vi "temperature_checksum.vi"(1 "Input string":string) -> (0 "Checksum":string)   [LabVIEW 2011]
doc: "moreChemistry's general purpose CRC vi\ncopyright 2004 moreChemistry BART BOSHUIZEN"
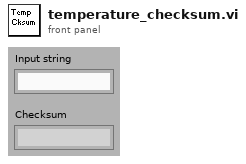
[diagram p1: front panel]
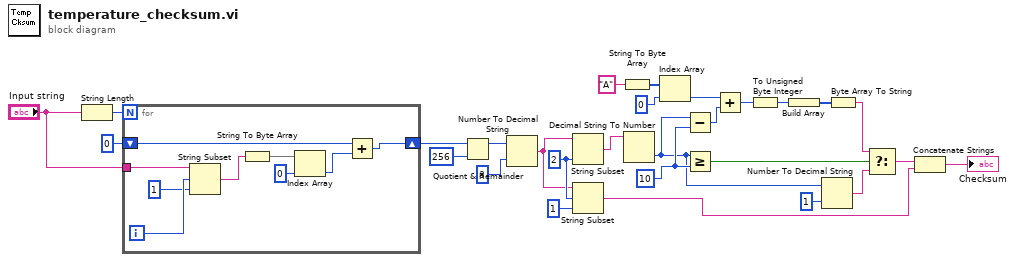
[diagram p0: block diagram]
diagram:
  w16 = 10 ("y")
  w8 = 2 ("length (rest)")
  n1 = String Length(string="Input string") -> (length=w25:i32)
  n2 = for {
    N: w25 -> [_]
    tunnel: "Input string" -> [w37]
    shift-right: [w32] -> w2
    shift-left: i16 0 -> [w30]
    i -> [w36]
    n3 = String Subset(string=w37, offset (0)=w36, length (rest)=1) -> (substring=w34:string)
    n4 = String To Byte Array(string=w34) -> (unsigned byte array=w31:u8[])
    n5 = Index Array(array=w31, index=0) -> (element=w29:u8)
    n6 = Add(x=w30, y=w29) -> (x+y=w32:i16)
  }
  n7 = Quotient & Remainder(x=w2, y=256) -> (x-y*floor(x/y)=w1:i32)  [unwired: 1 out]
  n8 = Number To Decimal String(number=w1, width (-)=i16 3) -> (decimal integer string=w6:string)
  n9 = String Subset(string=w6, length (rest)=w8) -> (substring=w23:string)  [unwired: 1 out]
  n10 = String Subset(string=w6, offset (0)=w8, length (rest)=1 ("length (rest)")) -> (substring=w4:string)
  n11 = String To Byte Array(string="A") -> (unsigned byte array=w18:u8[])
  n12 = Decimal String To Number(string=w23) -> (number=w12:i32)  [unwired: 3 out]
  n13 = Index Array(array=w18, index=0) -> (element=w14:u8)
  n14 = Subtract(x=w12, y=w16) -> (x-y=w15:i32)
  n15 = Greater Or Equal?(x=w12, y=w16) -> (x >= y?=w22:bool)
  n16 = Add(x=w14, y=w15) -> (x+y=w13:i32)
  n17 = To Unsigned Byte Integer(number=w13) -> (unsigned 8bit integer=w21:u8)
  n18 = Build Array(w21) -> (w20:u8[])
  n19 = Number To Decimal String(number=w12, width (-)=i16 1) -> (decimal integer string=w9:string)
  n20 = Byte Array To String(unsigned byte array=w20) -> (string=w10:string)
  n21 = Select(t=w10, s=w22, f=w9) -> (s? t:f=w5:string)
  n22 = Concatenate Strings(w5, w4) -> (→"Checksum":string)
